vi "Prompt for Custom Filter.vi"(6 "Calling VI in":refnum<vi>, 8 "error in (no error)":errorcluster, 11 "Filter Info":T1={"Filter Column"=enum."Description", "Filter Type"=enum."Contains", "Filter Value"="", "New Data?"=FALSE, "Enabled?"=FALSE}) -> (0 "error out":errorcluster, 2 "OK?":bool, 3 "Filter Info out":T1={"Filter Column"=enum."Description", "Filter Type"=enum."Contains", "Filter Value"="", "New Data?"=FALSE, "Enabled?"=FALSE})   [LabVIEW 2023, in "VI Properties Editor.lvlib"]
doc: "Displays a window to add a custom filter."
uses:
  VI Properties Editor.lvlib
  CTLs/Column Name.ctl
  CTLs/Filter Type.ctl
  CTLs/Filter Info.ctl
panel:
  in  "Cancel":bool
  in  "OK":bool
  in  "Filter Type Enum":T3
  in  "Filter Type":u16(ring) items=["Contains", "Equals", "Starts with", "Ends with", "Does not contain", "Does not equal", "Is empty", "Is not empty"]
  in  "Filter Column":u16(ring) items=["Name", "Path", "Type", "Window Title", "Description", "Help Path", "Help Tag", "Custom Title?", "Reentrant?", "Inlined?"]
  in  "Filter Value":string
  in  "Filter Column Enum":T2
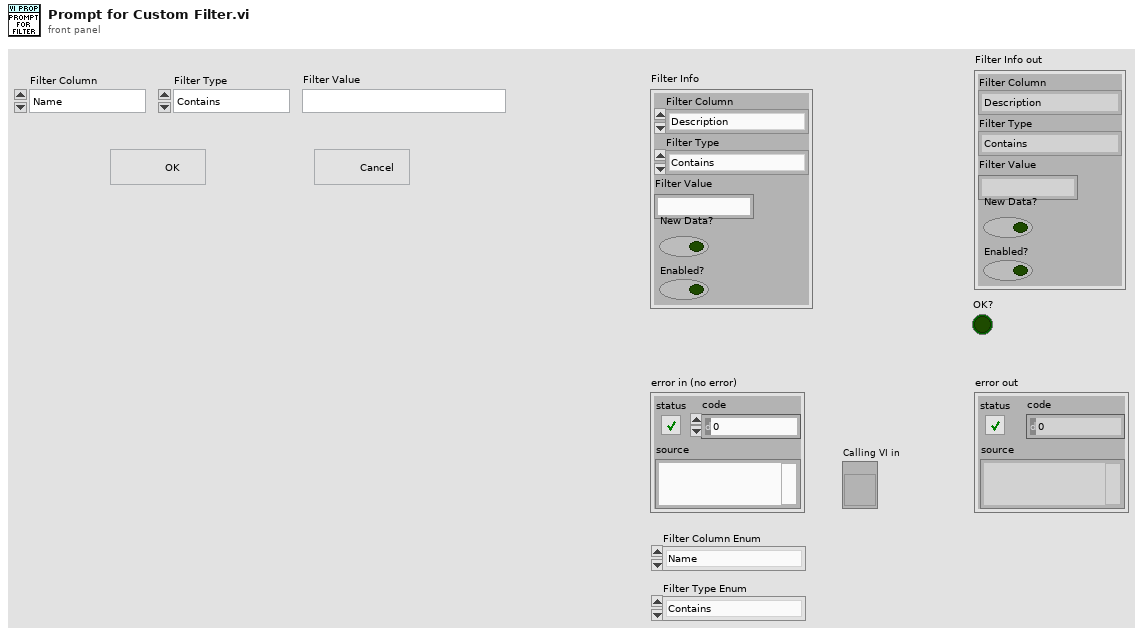
[diagram p1: front panel]
types:
  T1 = typedef "VI Properties Editor.lvlib/Filter Info.ctl" = cluster{"Filter Column":T2, "Filter Type":T3, "Filter Value":string, "New Data?":bool, "Enabled?":bool}
  T2 = typedef "VI Properties Editor.lvlib/Column Name.ctl" = enum16{"Name", "Path", "Type", "Window Title", "Description", "Help Path", "Help Tag", "Custom Title?", "Reentrant?", "Inlined?"}
  T3 = typedef "VI Properties Editor.lvlib/Filter Type.ctl" = enum16{"Contains", "Equals", "Starts with", "Ends with", "Does not contain", "Does not equal", "Is empty", "Is not empty"}
  T4 = enum32{"Invalid", "Standard", "Closed", "Hidden", "Minimized", "Maximized"}
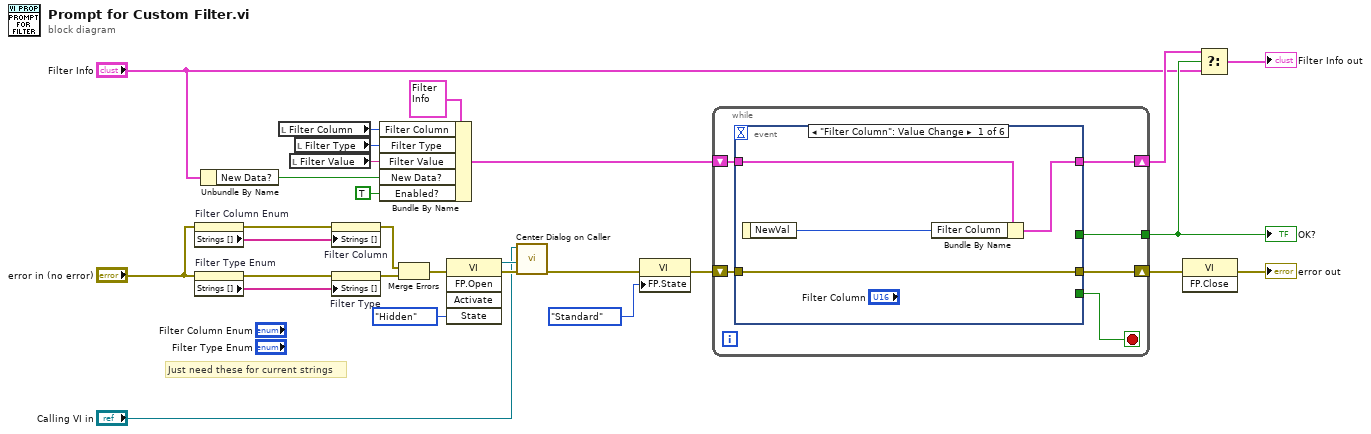
[diagram p0: block diagram]
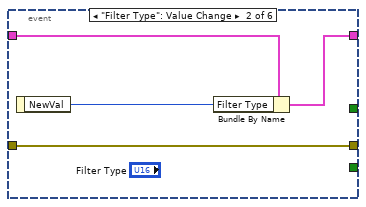
[diagram p2: hidden frame]
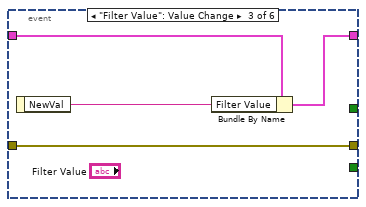
[diagram p3: hidden frame]
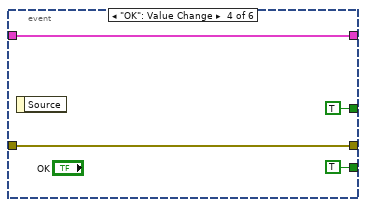
[diagram p4: hidden frame]
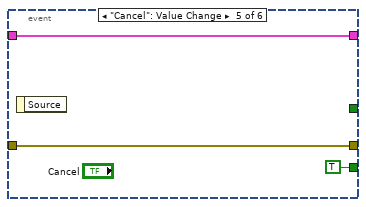
[diagram p5: hidden frame]
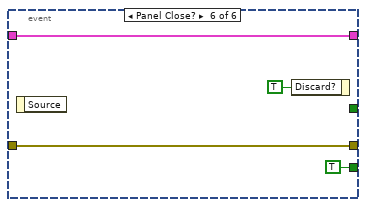
[diagram p6: hidden frame]
diagram:
  # "Just need these for current strings"
  n1 = property on="Filter Column Enum" class="Enum (strict)"(error in="error in (no error)") -> (error out=w26:errorcluster, "Strings []"=w28:string[])  [unwired: 1 in, 1 out]
  n2 = property on="Filter Type Enum" class="Enum (strict)"(error in="error in (no error)") -> (error out=w25:errorcluster, "Strings []"=w27:string[])  [unwired: 1 in, 1 out]
  n3 = Unbundle By Name("Filter Info") -> ("New Data?"=w9:bool)
  n4 = local read "Filter Column"() -> (w12:u16)
  n5 = local read "Filter Value"() -> (w13:string)
  n6 = local read "Filter Type"() -> (w11:u16)
  n7 = property on="Filter Column" class="Ring (strict)"(error in=w26, "Strings []"=w28) -> (error out=w24:errorcluster)  [unwired: 1 in, 1 out]
  n8 = property on="Filter Type" class="Ring (strict)"(error in=w25, "Strings []"=w27) -> (error out=w23:errorcluster)  [unwired: 1 in, 1 out]
  n9 = Bundle By Name(cluster=T1 {"Filter Column"=enum."Description", "Filter Type"=enum."Contains", "Filter Value"="", "New Data?"=FALSE, "Enabled?"=FALSE} ("Filter Info"), "Filter Column"=w12, "Filter Type"=w11, "Filter Value"=w13, "New Data?"=w9, "Enabled?"=TRUE) -> (w16:T1)
  n10 = Merge Errors(w24, w23) -> (w2:errorcluster)
  n11 = invoke class="VI" method="FP.Open"(error in=w2, "State"=T4."Hidden") -> (reference out=w5:refnum<vi>, error out=w6:errorcluster)  [unwired: 3 in, 3 out]
  n12 = call "Center Dialog on Caller.vi"("error in (no error)"=w6, "Dialog VI"=w5, "Calling VI in"="Calling VI in") -> ("error out"=w8:errorcluster)  [unwired: 7 in, 1 out]
  n13 = property class="VI"(error in=w8, "FP.State"=T4."Standard" ("Front Panel Window:State")) -> (error out=w1:errorcluster)  [unwired: 1 in, 1 out]
  n14 = while {
    tunnel: [w29] -> w19
    shift-right: [w33] -> w18
    shift-left: w16 -> [w34]
    shift-right: [w31] -> w22
    shift-left: w1 -> [w32]
    stop <- w30 stop-if-true
    n15 = event shown="[0] \"Filter Column\": Value Change" {
      selector: _ -> [_ _ _ _ _ _]
      dyn-events: _ -> [_ _ _ _ _ _]
      timeout: _ -> [_ _ _ _ _ _]
      tunnel: w34 -> [w38 w42 w46 w47 w51 w54]
      tunnel: [w36 w40 w44 w47 w51 w54] -> w33
      tunnel: w32 -> [w35 w39 w43 w50 w53 w57]
      tunnel: [w35 w39 w43 w50 w53 w57] -> w31
      tunnel: [_ _ _ TRUE TRUE TRUE] -> w30
      tunnel: [_ _ _ TRUE _ _] -> w29
      event "Filter Column": Value Change {
        n16 = event-data() -> ("NewVal"=w37:u16)  [unwired: 1 in]
        n17 = Bundle By Name(cluster=w38, "Filter Column"=w37) -> (w36:T1)
      }
      event "Filter Type": Value Change {
        n18 = event-data() -> ("NewVal"=w41:u16)  [unwired: 1 in]
        n19 = Bundle By Name(cluster=w42, "Filter Type"=w41) -> (w40:T1)
      }
      event "Filter Value": Value Change {
        n20 = event-data() -> ("NewVal"=w45:string)  [unwired: 1 in]
        n21 = Bundle By Name(cluster=w46, "Filter Value"=w45) -> (w44:T1)
      }
      event "OK": Value Change {
        n22 = event-data() -> ()  [unwired: 1 in, 1 out]
      }
      event "Cancel": Value Change {
        n23 = event-data() -> ()  [unwired: 1 in, 1 out]
      }
      event Panel Close? {
        n24 = event-data() -> ()  [unwired: 1 in, 1 out]
        n25 = event-data("Discard?"=TRUE) -> ()  [unwired: 1 in, 1 out]
      }
    }
  }
  "OK?" <- w19
  n26 = invoke class="VI" method="FP.Close"(error in=w22) -> (error out=→"error out":errorcluster)  [unwired: 2 in, 2 out]
  n27 = Select(t=w18, s=w19, f="Filter Info") -> (s? t:f=→"Filter Info out":T1)
